vi "Event Handler.vi"(0 "uService Template in":refnum<class "DAQ Sender.lvclass">, 5 "Event type":T1=enum."Message", 7 "Item Name":string, 9 "Data":variant, 11 "error in (no error)":errorcluster) -> (4 "uService Template out":refnum<class "DAQ Sender.lvclass">, 15 "error out":errorcluster)   [LabVIEW 2020, in "DAQ Sender.lvlib" / "DAQ Sender.lvclass"]
uses:
  DAQ Sender.lvclass
  C:/Users/marco/Documents/GitHub_Lab/TALOS/talos/Father of all uServices/Father of all uServices/Father of all uServices.lvclass
  Father of all uServices/Father of all uServices/Event Handler Items.ctl
  Ancestor/Ancestor/Ancestor.lvclass/Ancestor.ctl
  DAQ Sender Consumer Case Selector.ctl
  Father of all uServices/Father of all uServices Messages/Consumer Msg/Consumer Msg.lvclass/Consumer Msg.ctl
  FGV/Error Memory/Get Error Description.vi
  Support VIs/Get PC name.vi
  Ancestor/Ancestor/Read ID.vi
  Support VIs/Get Class Name.vi
  <vilib>/Utility/error.llb/Clear Errors.vi
  Father of all uServices/Father of all uServices Messages/Consumer Msg/Send Consumer.vi
  Support VIs/Substitute Error.vi
  FGV/Error Memory/Error Memory Core.vi
  <vilib>/AdvancedString/Delimited String to 1D String Array.vi
  Support VIs/Circus Root Path.vi
  FGV/Error Memory/Error Crt Lvl checker.vi
  FGV/Error Memory/Error Memory Core.vi/40c8088d-b597-4017-91af-faa98e00292e.vi
  FGV/Error Memory/Error Memory Core.vi/d4a3ab98-063c-4e44-b43d-fbdcfe6c2be2.vi
  Father of all uServices/Father of all uServices/Father of all uServices.lvclass
  C:/Users/marco/Documents/GitHub_Lab/TALOS/builds/Actor Framework PPL/Actor Framework.lvlibp/1abvi3w/vi.lib/ActorFramework/Actor/Actor.lvclass
  Support VIs/Global Memory.vi
  <vilib>/Utility/LVClass/Get LV Class Name.vi
  Support VIs/Is in Packed Library.vi
  Support VIs/TALOS Root path.vi
  Support VIs/Read CSV worksheet.vi
  Support VIs/Global Constants.vi
  <vilib>/Utility/error.llb/General Error Handler.vi
  builds/Actor Framework PPL/Actor Framework.lvlibp/1abvi3w/vi.lib/ActorFramework/Actor/Read Self Enqueuer.vi
  <userlib>/_OpenG.lib/lvdata/lvdata.llb/Get Strings from Enum__ogtk.vi
  builds/Actor Framework PPL/Actor Framework.lvlibp/1abvi3w/vi.lib/ActorFramework/Message Enqueuer/Enqueue.vi
  Support VIs/Error Log.vi
  Ancestor/Ancestor/Ancestor.lvclass
  <vilib>/Comparison/Equal/Equal Functor/Equal Functor.lvclass
  Father of all uServices/Father of all uServices Messages/Consumer Msg/Consumer Msg.lvclass
  TALOS.lvlib
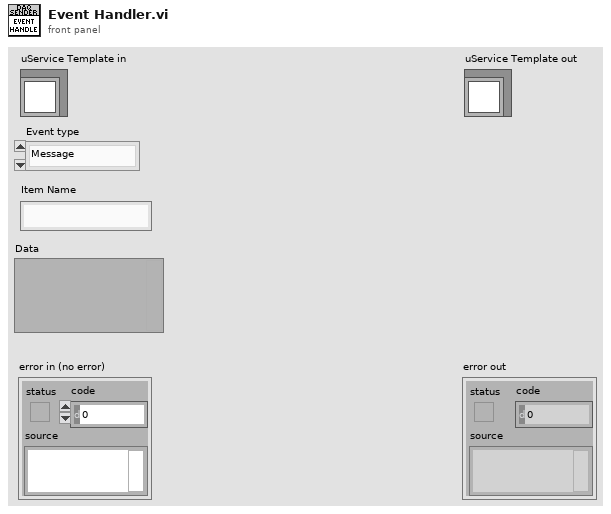
[diagram p1: front panel]
types:
  T1 = typedef "TALOS.lvlib/Father of all uServices.lvlib/Father of all uServices.lvclass/Event Handler Items.ctl" = enum16{"Button Pressed", "Shared Variable Updated", "Message", "Ready to launch?", "Safe Mode", "Start RUN", "Stop RUN"}
  T2 = typedef "DAQ Sender.lvlib/DAQ Sender.lvclass/DAQ Sender Consumer Case Selector.ctl" = enum16{"Send to DAQ"}
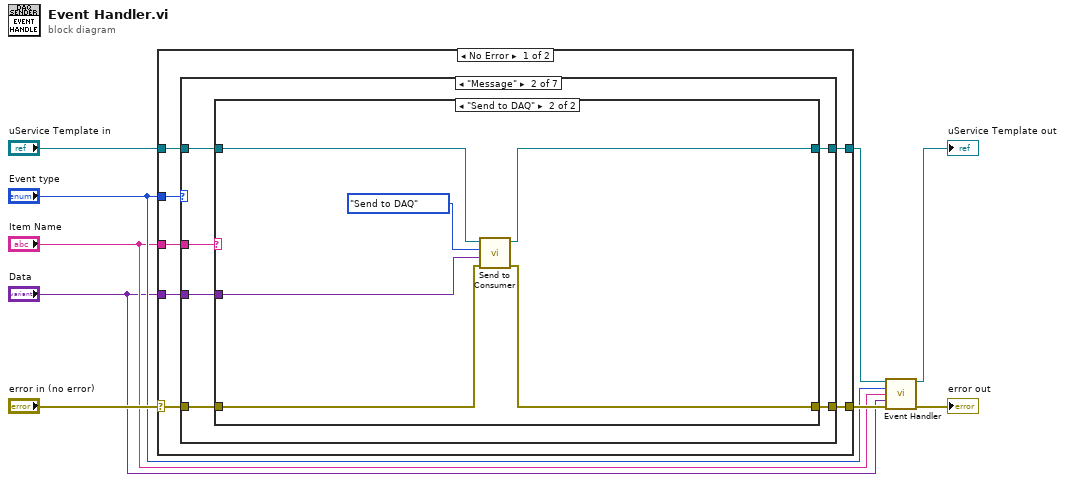
[diagram p0: block diagram]
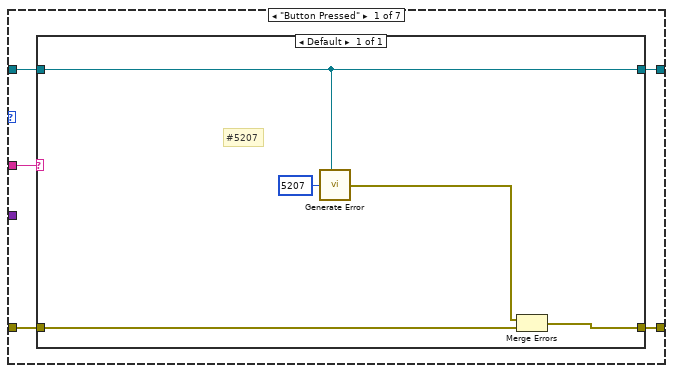
[diagram p2: hidden frame]
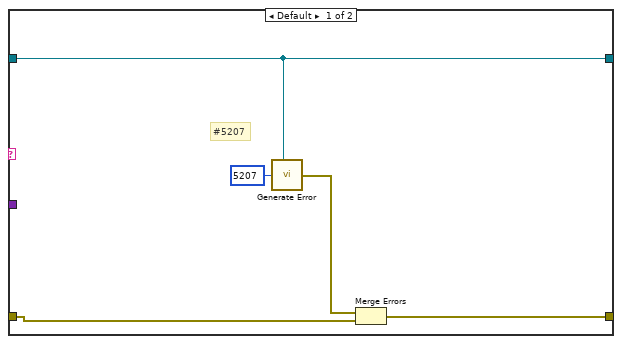
[diagram p3: hidden frame]
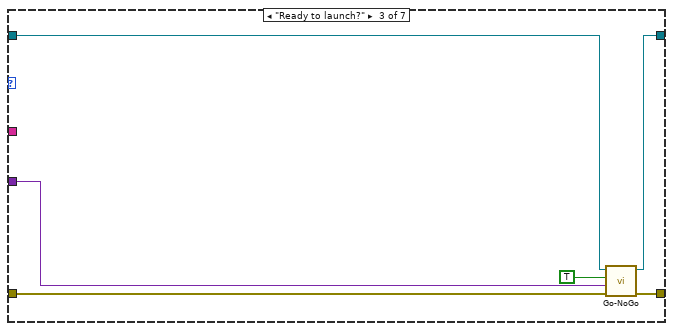
[diagram p4: hidden frame]
diagram:
  n1 = case shown="No Error" "error in (no error)" {
    selector: "error in (no error)" -> [w13 w59]
    tunnel: [w12 w59] -> w7
    tunnel: "uService Template in" -> [w15 w58]
    tunnel: [w14 w58] -> w4
    tunnel: "Event type" -> [w16 _]
    tunnel: "Item Name" -> [w11 _]
    tunnel: "Data" -> [w10 _]
    frame No Error {
      n2 = case shown="\"Message\"" w16 {
        tunnel: w15 -> [w21 w32 w46 w51 w53 w55 w57]
        tunnel: [w20 w28 w49 w51 w53 w55 w57] -> w14
        tunnel: w13 -> [w17 w29 w47 w50 w52 w54 w56]
        tunnel: [w18 w27 w48 w50 w52 w54 w56] -> w12
        tunnel: w11 -> [w19 w31 _ _ _ _ _]
        tunnel: w10 -> [_ w30 w44 _ _ _ _]
        frame "Button Pressed" {
          n3 = case shown="Default" w19 {
            tunnel: w21 -> [w22]
            tunnel: [w22] -> w20
            tunnel: [w25] -> w18
            tunnel: w17 -> [w26]
            frame Default {
              # "#5207"
              n4 = call "Generate Error.vi"("Class"=w22, "Error Code"=5207) -> ("error out"=w24:errorcluster)  [unwired: 5 in]
              n5 = Merge Errors(w24, w26) -> (w25:errorcluster)
            }
          }
        }
        frame "Message" {
          n6 = case shown="\"Send to DAQ\"" w31 {
            tunnel: w32 -> [w35 w43]
            tunnel: w30 -> [_ w38]
            tunnel: w29 -> [w33 w41]
            tunnel: [w35 w39] -> w28
            tunnel: [w34 w40] -> w27
            frame Default {
              # "#5207"
              n7 = call "Generate Error.vi"("Class"=w35, "Error Code"=5207) -> ("error out"=w36:errorcluster)  [unwired: 5 in]
              n8 = Merge Errors(w36, w33) -> (w34:errorcluster)
            }
            frame "Send to DAQ" {
              n9 = call "Send to Consumer.vi"("error in (no error)"=w41, "Data"=w38, "Case ID"=DAQ_Sender_Consumer_Case_Selector."Send to DAQ", "uService Template in"=w43) -> ("error out"=w40:errorcluster, "uService Template out"=w39:refnum<class "DAQ Sender.lvclass">)  [unwired: 6 in]
            }
          }
        }
        frame "Ready to launch?" {
          n10 = call-dynamic "Go-NoGo.vi"("error in (no error)"=w47, "Go-NoGo Data"=w44, "Go?"=TRUE, "Father of all uServices in"=w46) -> ("error out"=w48:errorcluster, "Father of all uServices out"=w49:refnum<class "DAQ Sender.lvclass">)  [unwired: 6 in]
        }
        frame "Safe Mode" {
        }
        frame "Start RUN" {
        }
        frame "Stop RUN" {
        }
        frame "Shared Variable Updated" {
        }
      }
    }
    frame Error {
    }
  }
  n11 = call-parent "Event Handler.vi"("uService Template in"=w4, "Event type"="Event type", "Item Name"="Item Name", "Data"="Data", "error in (no error)"=w7) -> ("uService Template out"=→"uService Template out":refnum<class "DAQ Sender.lvclass">, "error out"=→"error out":errorcluster)  [unwired: 9 in]
